vi "PPSU end string finder.vi"(8 "error in (no error)":errorcluster, 9 "stop":bool, 11 "TCP Network Connection in":refnum<k5>) -> (0 "error out":errorcluster, 2 "String":string, 3 "TCP Network Connection out":refnum<k5>)   [LabVIEW 2022 SP3]
panel:
  out "x-y":u32
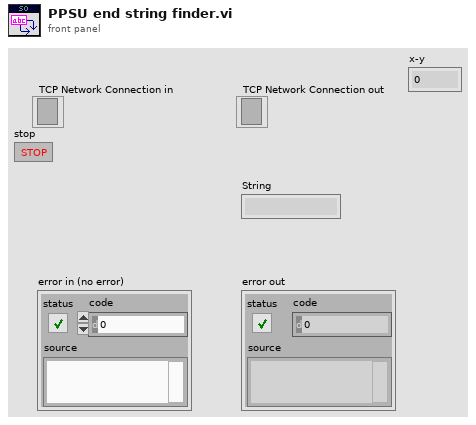
[diagram p1: front panel]
types:
  T1 = enum16{"Standard", "Buffered", "CRLF", "Immediate"}
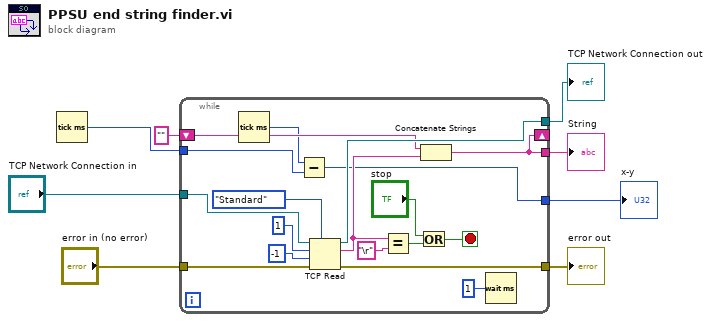
[diagram p0: block diagram]
diagram:
  n1 = Tick Count (ms)() -> (millisecond timer value=w2:u32)
  n2 = while {
    tunnel: [w15] -> w6
    tunnel: "error in (no error)" -> [w20]
    tunnel: [w25] -> w3
    tunnel: "TCP Network Connection in" -> [w21]
    tunnel: [w26] -> w8
    shift-right: [w15] -> _
    shift-left: "" -> [w16]
    tunnel: w2 -> [w10]
    tunnel: [w11] -> w1
    stop <- w13 stop-if-true
    n3 = Tick Count (ms)() -> (millisecond timer value=w9:u32)
    n4 = Subtract(x=w9, y=w10) -> (x-y=w11:u32)
    n5 = TCP Read(connection ID=w21, bytes to read=1, error in (no error)=w20, 7:T1."Standard" ("mode (standard)"), 9:-1 ("timeout ms (25000)")) -> (connection ID out=w26:refnum<k5>, data out=w18:string, error out=w25:errorcluster)
    n6 = Equal?(x=w18, y="\r") -> (x = y?=w14:bool)
    n7 = Or(x="stop", y=w14) -> (x .or. y?=w13:bool)
    n8 = Concatenate Strings(w16, w18) -> (w15:string)
    n9 = Wait (ms)(milliseconds to wait=u32 1) -> ()  [unwired: 1 out]
  }
  "TCP Network Connection out" <- w8
  "String" <- w6
  "error out" <- w3
  "x-y" <- w1
